vi "SLSC Set Item for Tree Control.vi"(9 "Modify Reset Value?":bool, 10 "Value":string, 11 "Item In":T1) -> (1 "Changed Column":i32, 3 "Item Out":T1)   [LabVIEW 2017, in "SLSC Tree Control.lvlib"]
doc: "Sets the default value or the reset value of the SLSC Tree Item."
uses:
  SLSC Tree Control.lvlib
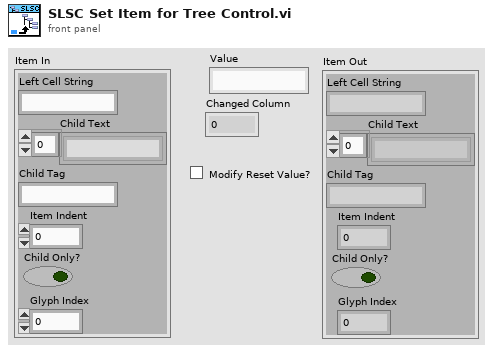
[diagram p1: front panel]
types:
  T1 = cluster{"Left Cell String":string, "Child Text":string[], "Child Tag":string, "Item Indent":i32, "Child Only?":bool, "Glyph Index":i32}
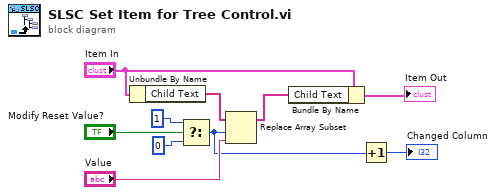
[diagram p0: block diagram]
diagram:
  n1 = Unbundle By Name("Item In") -> ("Child Text"=w8:string[])
  n2 = Select(t=1, s="Modify Reset Value?", f=0 ("index")) -> (s? t:f=w2:i32)
  n3 = Replace Array Subset(array=w8, new element="Value", index=w2) -> (w7:string[])
  n4 = Bundle By Name(cluster="Item In", "Child Text"=w7) -> (→"Item Out":T1)
  n5 = Increment(x=w2) -> (x+1=→"Changed Column":i32)
